vi "Signal Pulse.vi"(1 "Input":bool) -> (0 "Output":bool)   [LabVIEW 2013]
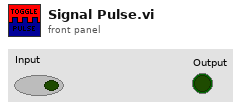
[diagram p1: front panel]
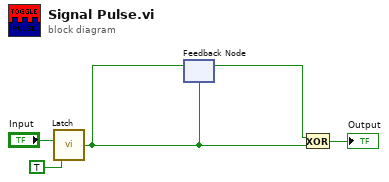
[diagram p0: block diagram]
diagram:
  n1 = call "Latch.vi"("Edge"=TRUE, "In"="Input") -> ("Out"=w1:bool)
  n2 = feedback-in #1(w1) -> ()
  n3 = feedback #1(w1) -> (w2:bool)
  n4 = Exclusive Or(1:w1, 2:w2) -> (0:→"Output":bool)
